vi "LIN USD Response.vi"(0 "DevHandle":i32, 1 "pRes":string, 5 "LINIndex":i32, 7 "ID":u8, 9 "NAD":u8, 11 "error in (no error)":errorcluster, 12 "pLen":u16) -> (3 "pRes out":string, 4 "function return":i32, 14 "pLen out":u16, 15 "error out":errorcluster)   [LabVIEW 2010, in "usb2lin_ex.lvlib"]
doc: "int WINAPI LIN_USD_Response(int DevHandle,int LINIndex,unsigned char ID,unsigned char NAD,unsigned char *pRes,unsigned short *pLen);"
uses:
  usb2lin_ex.lvlib
  USB2XXX.dll
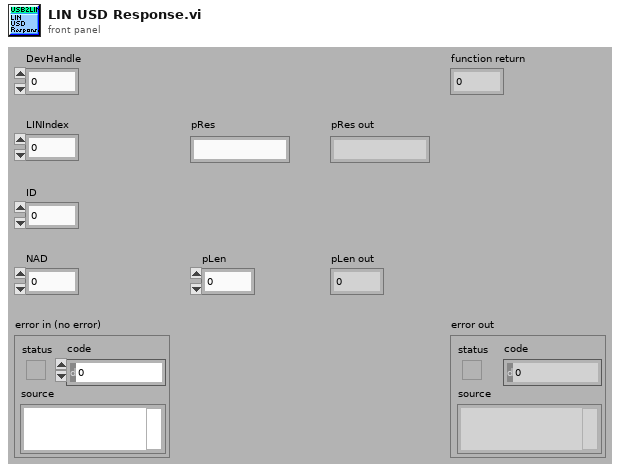
[diagram p1: front panel]
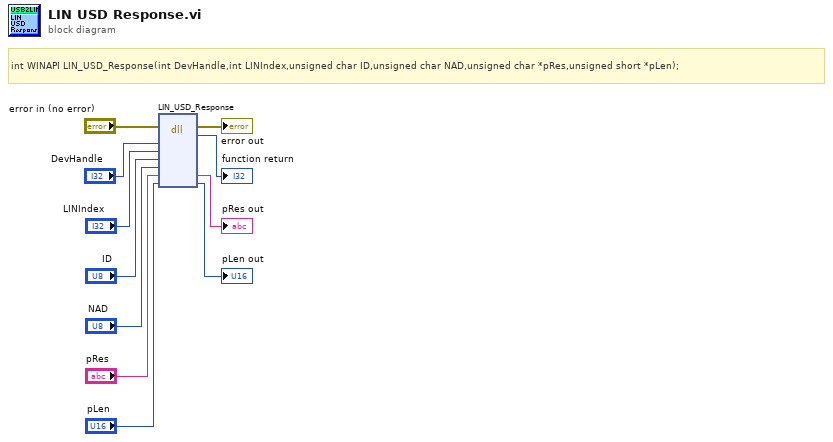
[diagram p0: block diagram]
diagram:
  # "int WINAPI LIN_USD_Response(int DevHandle,int LINIndex,unsigned char ID,unsigned char NAD,unsigned char *pRes,unsigned short *pLen);"
  n1 = dll-call lib="E:/OtherWork/STM32/USB2XXX_Example/sdk/api/Labview/USB2XXX.*" fn="LIN_USD_Response"(error in="error in (no error)", "DevHandle"="DevHandle", "LINIndex"="LINIndex", "ID"="ID", "NAD"="NAD", "pRes"="pRes", "pLen"="pLen") -> (error out=→"error out":errorcluster, →"function return":i32, "pRes"=→"pRes out":string, "pLen"=→"pLen out":u16)  [unwired: 6 in, 1 out]
